vi "Add_Log_File_comment_server.vi"(0 "Comments to Add to the Log files":string) -> ()   [LabVIEW 2010]
uses:
  ADAM_Global.vi
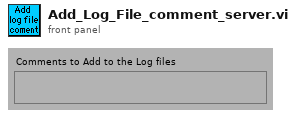
[diagram p1: front panel]
types:
  T1 = typedef "Comments_cluster.ctl" = cluster{"Time":dbl, "Comment":string}
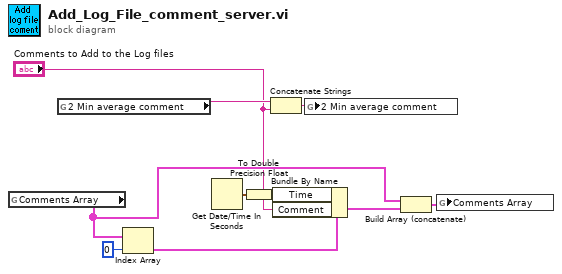
[diagram p0: block diagram]
diagram:
  n1 = global read "ADAM_Global.vi" "Comments Array"() -> (w5:T1[])
  n2 = global read "ADAM_Global.vi" "2 Min average comment"() -> (w10:string)
  n3 = Index Array(array=w5, index=0 ("Index")) -> (element=w7:T1)
  n4 = Get Date/Time In Seconds() -> (seconds since 1Jan1904=w1:timestamp)
  n5 = To Double Precision Float(number=w1) -> (double precision float=w6:dbl)
  n6 = Concatenate Strings(w10, "Comments to Add to the Log files") -> (w9:string)
  n7 = Bundle By Name(cluster=w7, "Time"=w6, "Comment"="Comments to Add to the Log files") -> (w4:T1)
  n8 = global write "ADAM_Global.vi" "2 Min average comment"(w9) -> ()
  n9 = Build Array (concatenate)(w5, w4) -> (w3:T1[])
  n10 = global write "ADAM_Global.vi" "Comments Array"(w3) -> ()
